vi "load_scope_config.vi"(7 "Load File Type":u16(ring) items=["Automatic Load", "Custom File"], 8 "error in":errorcluster, 9 "Controls References Cluster In":T1, 10 "Controls cluster":T5 {"C1 vertical coupling / V" items=["AC", "DC", "Ground"]; "C2 vertical coupling / V" items=["AC", "DC", "Ground"]; "Trigger slope" items=["Positive", "Negative"]}, 11 "Current VI's Path":path=path "" caption="start path") -> (0 "error out":errorcluster, 1 "Controls References Cluster Out":T1, 2 "Controls cluster out":T5 {"C1 vertical coupling / V" items=["AC", "DC", "Ground"]; "C2 vertical coupling / V" items=["AC", "DC", "Ground"]; "Trigger slope" items=["Positive", "Negative"]})   [LabVIEW 2023]
uses:
  <instrlib>/niScope/Controls/niScope vertical coupling.ctl
  <instrlib>/niScope/Controls/niScope trigger source.ctl
  <instrlib>/niScope/Controls/niScope trigger slope.ctl
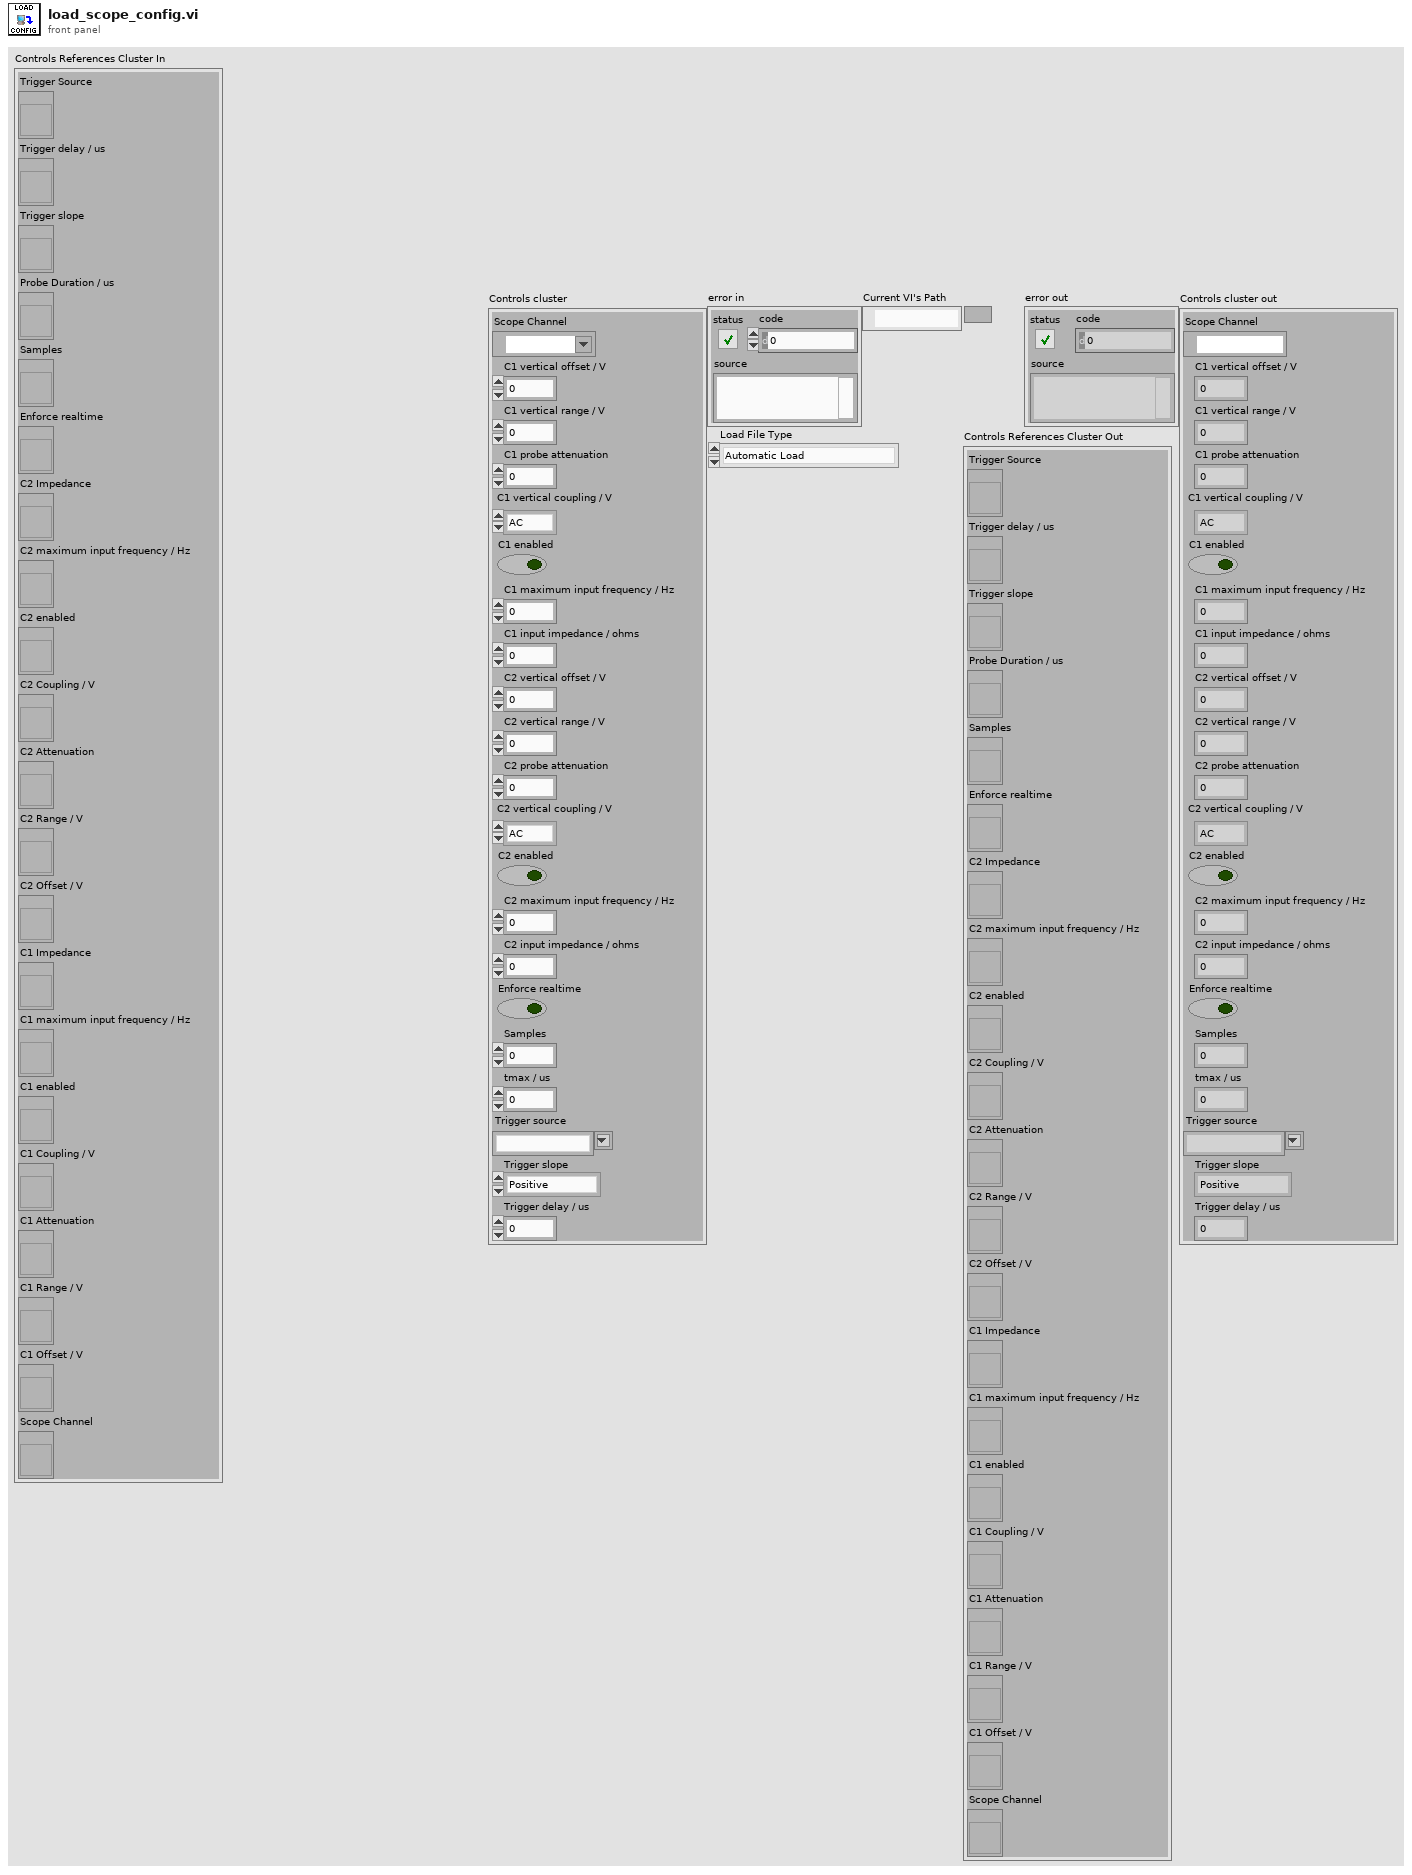
[diagram p1: front panel]
types:
  T1 = cluster{"Trigger Source":refnum<vi>, "Trigger delay / us":refnum<vi>, "Trigger slope":refnum<vi>, "Probe Duration / us":refnum<vi>, "Samples":refnum<vi>, "Enforce realtime":refnum<vi>, "C2 Impedance":refnum<vi>, "C2 maximum input frequency / Hz":refnum<vi>, "C2 enabled":refnum<vi>, "C2 Coupling / V":refnum<vi>, "C2 Attenuation":refnum<vi>, "C2 Range / V":refnum<vi>, "C2 Offset / V":refnum<vi>, "C1 Impedance":refnum<vi>, "C1 maximum input frequency / Hz":refnum<vi>, "C1 enabled":refnum<vi>, "C1 Coupling / V":refnum<vi>, "C1 Attenuation":refnum<vi>, "C1 Range / V":refnum<vi>, "C1 Offset / V":refnum<vi>, "Scope Channel":refnum<vi>}
  T2 = typedef "niScope vertical coupling.ctl" = i32
  T3 = typedef "niScope trigger source.ctl" = string
  T4 = typedef "niScope trigger slope.ctl" = i32
  T5 = cluster{"Scope Channel":refnum<k15>, "C1 vertical offset / V":dbl, "C1 vertical range / V":dbl, "C1 probe attenuation":dbl, "C1 vertical coupling / V":T2, "C1 enabled":bool, "C1 maximum input frequency / Hz":dbl, "C1 input impedance / ohms":u32, "C2 vertical offset / V":dbl, "C2 vertical range / V":dbl, "C2 probe attenuation":dbl, "C2 vertical coupling / V":T2, "C2 enabled":bool, "C2 maximum input frequency / Hz":dbl, "C2 input impedance / ohms":u32, "Enforce realtime":bool, "Samples":i64, "tmax / us ":dbl, "Trigger source":T3, "Trigger slope":T4, "Trigger delay / us":dbl}
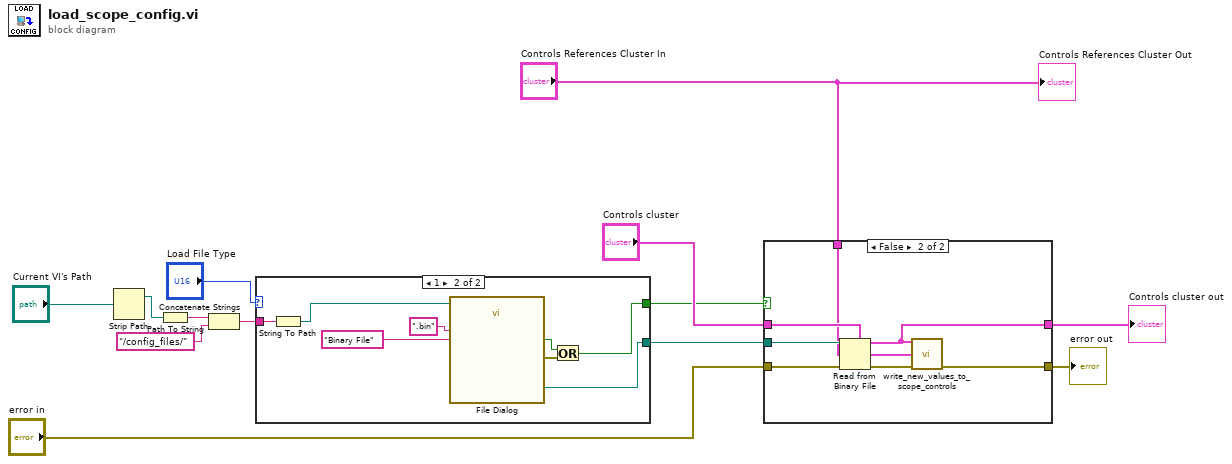
[diagram p0: block diagram]
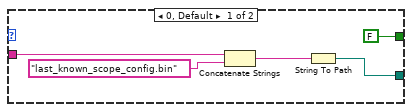
[diagram p2: hidden frame]
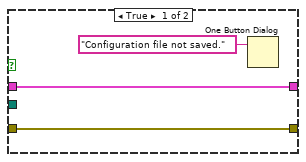
[diagram p3: hidden frame]
diagram:
  n1 = Strip Path(path="Current VI's Path") -> (stripped path=w6:path)  [unwired: 1 out]
  n2 = Path To String(path=w6) -> (string=w5:string)
  n3 = Concatenate Strings(w5, "/config_files/" ("string")) -> (w3:string)
  n4 = case shown="1" "Load File Type" {
    tunnel: [FALSE w22] -> w8
    tunnel: [w15 w21] -> w7
    tunnel: w3 -> [w18 w20]
    frame 0, Default {
      n5 = Concatenate Strings(w18, "last_known_scope_config.bin" ("string")) -> (w16:string)
      n6 = String To Path(string=w16) -> (path=w15:path)
    }
    frame 1 {
      n7 = String To Path(string=w20) -> (path=w19:path)
      n8 = call "File Dialog"("start path"=w19, "pattern (all files)"=".bin", "pattern label"="Binary File") -> ("selected path"=w21:path, "cancelled"=w26:bool, "error out"=w25:errorcluster)  [unwired: 9 in, 1 out]
      n9 = Or(x=w26, y=w25) -> (x .or. y?=w22:bool)
    }
  }
  n10 = case shown="False" w8 {
    tunnel: "Controls cluster" -> [w28 w31]
    tunnel: "error in" -> [w29 w36]
    tunnel: [w29 w32] -> w11
    tunnel: w7 -> [_ w35]
    tunnel: [w28 w34] -> w10
    tunnel: "Controls References Cluster In" -> [_ w30]
    frame True {
      n11 = One Button Dialog(message="Configuration file not saved.") -> ()  [unwired: 1 in, 1 out]
    }
    frame False {
      n12 = Read from Binary File(5:w31, 8:w36, 11:w35) -> (0:w33:errorcluster, 2:w34:T5)  [unwired: 3 in, 2 out]
      n13 = call "write_new_values_to_scope_controls.vi"("Controls Cluster"=w34, "Controls References Cluster"=w30, "error in (no error)"=w33) -> ("error out"=w32:errorcluster)  [unwired: 12 in]
    }
  }
  "error out" <- w11
  "Controls cluster out" <- w10
  "Controls References Cluster Out" <- "Controls References Cluster In"
